vi "Find Job On Other Machines.vi"(7 "Job Schedule on Machines":i32[][](array[numeric]), 8 "Number of Machines":i32, 9 "Machine No":i32, 10 "Job No":i32, 11 "Gannt Chart":T2[][](array[typedef])) -> (2 "Time Interval List":T1[](array[typedef]))   [LabVIEW 2013, in "Scheduler.lvclass"]
uses:
  Scheduler.lvclass
  Controls/GanntChart_Element.ctl
  Controls/Time_Interval_List_Element.ctl
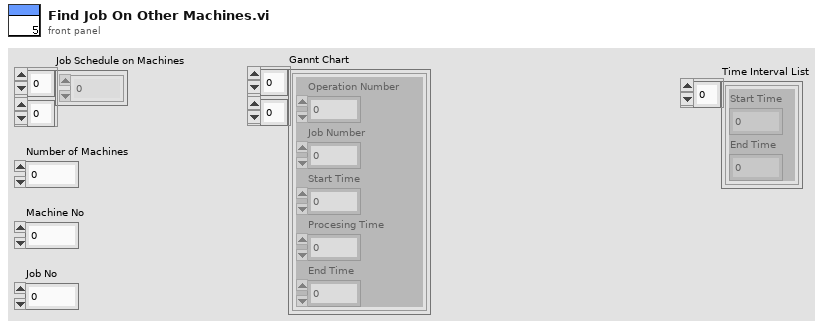
[diagram p1: front panel]
types:
  T1 = typedef "Time_Interval_List_Element.ctl" = cluster{"Start Time":i32, "End Time":i32}
  T2 = typedef "GanntChart_Element.ctl" = cluster{"Operation Number":i32, "Job Number":i32, "Start Time":i32, "Procesing Time":u16, "End Time":i32}
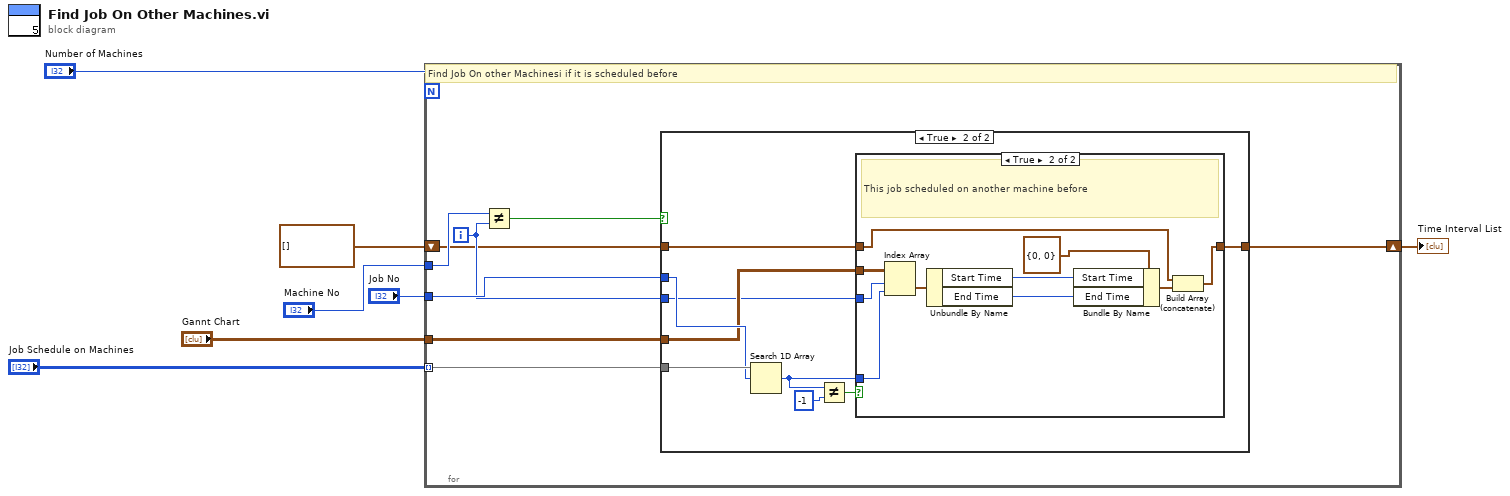
[diagram p0: block diagram]
diagram:
  n1 = for {
    N: "Number of Machines" -> [_]
    tunnel: "Machine No" -> [w13]
    tunnel: "Job No" -> [w14]
    tunnel: "Job Schedule on Machines" -> [w15] mode=indexing
    tunnel: "Gannt Chart" -> [w11]
    shift-right: [w8] -> w3
    shift-left: T1[] [] -> [w9]
    i -> [w10]
    # "Find Job On other Machinesi if it is scheduled before"
    n2 = Not Equal?(x=w13, y=w10) -> (x != y?=w12:bool)
    n3 = case shown="True" w12 {
      tunnel: w15 -> [_ w25]
      tunnel: w14 -> [_ w24]
      tunnel: w11 -> [_ w21]
      tunnel: w10 -> [_ w20]
      tunnel: w9 -> [w16 w18]
      tunnel: [w16 w17] -> w8
      frame False {
      }
      frame True {
        n4 = Search 1D Array(1D array=w25, element=w24) -> (index of element=w19:i32)  [unwired: 1 in]
        n5 = Not Equal?(x=w19, y=-1) -> (x != y?=w22:bool)
        n6 = case shown="True" w22 {
          tunnel: w21 -> [_ w36]
          tunnel: w20 -> [_ w35]
          tunnel: w19 -> [_ w34]
          tunnel: w18 -> [w26 w32]
          tunnel: [w26 w27] -> w17
          frame False {
          }
          frame True {
            # "This job scheduled on another machine before"
            n7 = Index Array(array=w36, index (row)=w35, index (col)=w34) -> (element=w33:T2)
            n8 = Unbundle By Name(w33) -> ("Start Time"=w30:i32, "End Time"=w29:i32)
            n9 = Bundle By Name(cluster=T1 {"Start Time"=0, "End Time"=0}, "Start Time"=w30, "End Time"=w29) -> (w28:T1)
            n10 = Build Array (concatenate)(w32, w28) -> (w27:T1[])
          }
        }
      }
    }
  }
  "Time Interval List" <- w3
